vi "Compute Histogram Thirds Standard Deviations.vi"(8 "Error In":errorcluster, 9 "Peak Positions":dbl[](array[numeric]), 10 "Y Array":dbl[](array[numeric]), 11 "X Array":dbl[](array[numeric])) -> (0 "Error Out":errorcluster, 3 "SDV Array":dbl[](array[numeric]))   [LabVIEW 2021, in "Histogram Window.lvlib"]
uses:
  Histogram Window.lvlib
  <userlib>/_OpenG.lib/array/array.llb/Sort 1D Array (DBL)__ogtk.vi
  <userlib>/_OpenG.lib/array/array.llb/openg_array.lvlib
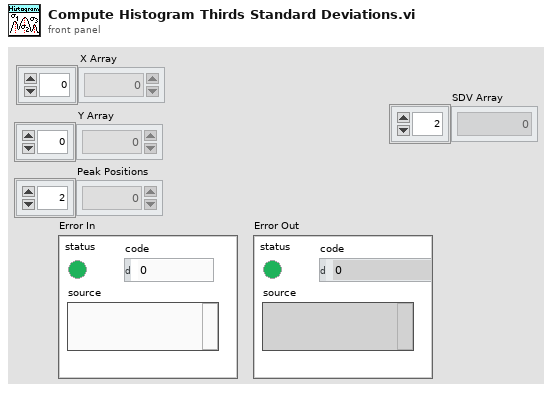
[diagram p1: front panel]
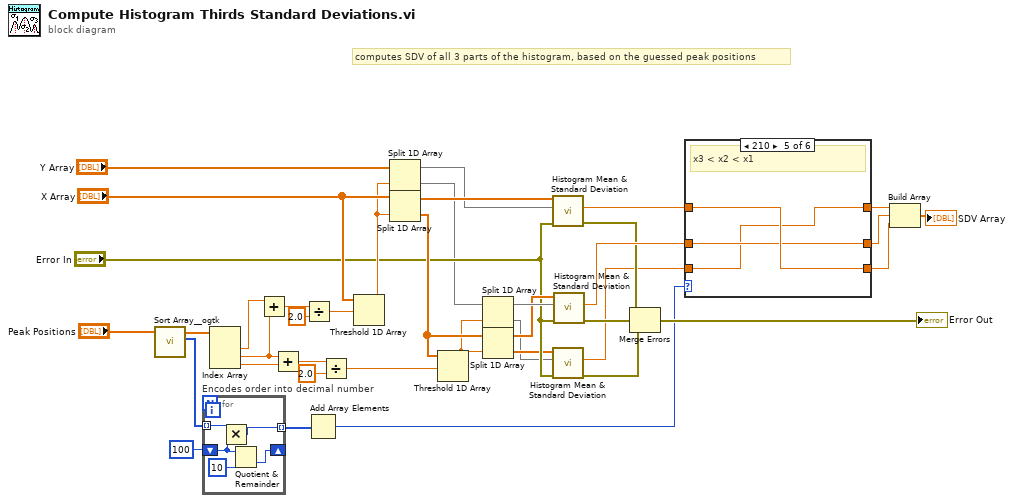
[diagram p0: block diagram]
diagram:
  # "computes SDV of all 3 parts of the histogram, based on the guessed peak positions"
  n1 = call-poly <userlib>:"Sort Array__ogtk.vi"("Array in"="Peak Positions") -> ("Sorted Pointers"=w9:i32[], "Sorted Array out"=w10:dbl[])  [unwired: 9 in]
  n2 = for "Encodes order into decimal number" {
    tunnel: w9 -> [w44] mode=indexing
    shift-right: [w41] -> _
    shift-left: 100 ("Numeric") -> [w42]
    tunnel: [w43] -> w7 mode=indexing
    n3 = Multiply(x=w44, y=w42) -> (x*y=w43:i32)
    n4 = Quotient & Remainder(x=w42, y=10 ("value")) -> (floor(x/y)=w41:i32)  [unwired: 1 out]
  }
  n5 = Index Array(array=w10) -> (element #1=w26:dbl, element #2=w25:dbl, element #3=w24:dbl)  [unwired: 3 in]
  n6 = Add(x=w26, y=w25) -> (x+y=w39:dbl)
  n7 = Add(x=w25, y=w24) -> (x+y=w23:dbl)
  n8 = Divide(x=w39, y=2.0) -> (x/y=w37:dbl)
  n9 = Add Array Elements(numeric array=w7) -> (sum=w6:i32)
  n10 = Divide(x=w23, y=2.0) -> (x/y=w21:dbl)
  n11 = Threshold 1D Array(2:w37, 3:"X Array") -> (0:w34:dbl)  [unwired: 1 in]
  n12 = Split 1D Array(array="Y Array", index=w34) -> (first subarray=w20:dbl[], second subarray=w1:dbl[])
  n13 = Split 1D Array(array="X Array", index=w34) -> (first subarray=w33:dbl[], second subarray=w19:dbl[])
  n14 = Threshold 1D Array(2:w21, 3:w19) -> (0:w18:dbl)  [unwired: 1 in]
  n15 = Split 1D Array(array=w1, index=w18) -> (first subarray=w17:dbl[], second subarray=w13:dbl[])
  n16 = Split 1D Array(array=w19, index=w18) -> (first subarray=w16:dbl[], second subarray=w14:dbl[])
  n17 = call "Histogram Mean & Standard Deviation.vi"("Error In"="Error In", "Histogram"=w20, "Values"=w33) -> ("Error Out"=w28:errorcluster, "Standard Deviation"=w32:dbl)  [unwired: 5 in, 2 out]
  n18 = call "Histogram Mean & Standard Deviation.vi"("Error In"="Error In", "Histogram"=w13, "Values"=w14) -> ("Error Out"=w11:errorcluster, "Standard Deviation"=w12:dbl)  [unwired: 5 in, 2 out]
  n19 = call "Histogram Mean & Standard Deviation.vi"("Error In"="Error In", "Histogram"=w17, "Values"=w16) -> ("Error Out"=w29:errorcluster, "Standard Deviation"=w30:dbl)  [unwired: 5 in, 2 out]
  n20 = Merge Errors(w28, w29, w11) -> (→"Error Out":errorcluster)
  n21 = case shown="210" w6 {
    tunnel: w32 -> [w47 w50 w53 w56 w59 w62]
    tunnel: [w46 w49 w53 w55 w57 w62] -> w31
    tunnel: w30 -> [w46 w49 w52 w55 w58 w61]
    tunnel: [w47 w48 w51 w56 w58 w61] -> w3
    tunnel: w12 -> [w45 w48 w51 w54 w57 w60]
    tunnel: [w45 w50 w52 w54 w59 w60] -> w2
    frame 120 {
      # "x2 < x3 < x1"
    }
    frame 201 {
      # "x3 < x1 < x2"
    }
    frame 21 {
      # "x1 < x3 < x2"
    }
    frame 102 {
      # "x2 < x1 < x3"
    }
    frame 210 {
      # "x3 < x2 < x1"
    }
    frame 12, Default {
      # "x1 < x2 < x3"
    }
  }
  n22 = Build Array(w31, w3, w2) -> (→"SDV Array":dbl[])
